vi "QuickTester.vi"() -> ()   [LabVIEW 2018]
uses:
  Real-Time/Control Algorithm/Control Algorithm Selection.ctl
  <vilib>/userdefined/High Color/nirio_resource_hc.ctl
  <vilib>/Simulation/Scripting/Companion Diagram/SimConfigNode/SimParams.ctl
  <vilib>/Simulation/Scripting/Companion Diagram/SimConfigNode/_simSolvers.ctl
  <vilib>/Simulation/Implementation/Shared/SIMSCR Execution Mode.ctl
  <vilib>/Platform/TimedLoop/XDataNode/timing_clust.ctl
  <vilib>/Platform/TimedLoop/XDataNode/nitl_modes.ctl
  <vilib>/Platform/TimedLoop/XDataNode/wakeup.ctl
  <vilib>/Simulation/Param Hierarchy/Typedefs/SIMPH Param Control Actions.ctl
  <vilib>/Simulation/Implementation/Shared/NILVSim_ParamChanged.vi
  <vilib>/Simulation/Implementation/Shared/NILVSim_FinishedLate.vi
  <vilib>/Simulation/Implementation/Shared/NILVSIM_BeginStep.vi
  <vilib>/Simulation/DiscreteLinear/Implementation/NILVSim Discrete State Space Direct.llb/SIM Discrete State Space Direct (MIMO).vi
  <vilib>/Simulation/Utility/Implementation/SIM Halt.vi
  <vilib>/Simulation/DiscreteLinear/Implementation/NILVSim Discrete Delay.llb/NILVSim Discrete Delay Buffered Distributor (scalar).vi
  <vilib>/Simulation/DiscreteLinear/Implementation/NILVSim Discrete Delay.llb/NILVSim Discrete Delay Buffered Collector (scalar).vi
  <vilib>/Simulation/Implementation/Shared/NILVSim_Manager.vi
  <vilib>/Utility/error.llb/Clear Errors.vi
  <vilib>/Simulation/Implementation/Shared/NILVSim_FinalizeModel.vi
  <vilib>/Simulation/Implementation/Shared/SIM Unbundle Sim Info.vi
  <vilib>/Simulation/Implementation/Shared/SIMSH Read Queue.vi
  <vilib>/Simulation/Implementation/Shared/NILVSim_Initialize.vi
  Real-Time/RT-FPGA Interface API/Read Tank Levels.vi
  <vilib>/Simulation/Utility/Implementation/NILVSim Get Time and IsAcceptedStep.vi
  <vilib>/Simulation/Implementation/Shared/NILVSim_GetModelError.vi
  <vilib>/Simulation/Implementation/Shared/SIM Bundle Sim Info.vi
  <vilib>/Simulation/Scripting/Companion Diagram/SimConfigNode/SimDog.xnode
  <vilib>/Platform/TimedLoop/XDataNode/XDataNode.xnode
  <vilib>/Simulation/Implementation/XNodeFramework/SimXNode/SimX.xnode
  Real-Time/RT-FPGA Interface API/RT-FPGA Interface API.lvlib
  <vilib>/Simulation/DiscreteLinear/Implementation/NILVSim Discrete Delay.llb/SIM Discrete Delay Buffered (scalar).vi
  <vilib>/Platform/TimedLoop/XDataNode/XDNodeRunTimeDep.lvlib
  <vilib>/Simulation/Implementation/Shared/NI_SIM_Implementation.lvlib
panel:
  out "coerced(x)":dbl[](array[numeric])
  in  "Halt?":bool
  out "Tanks levels":dbl[](array[numeric])
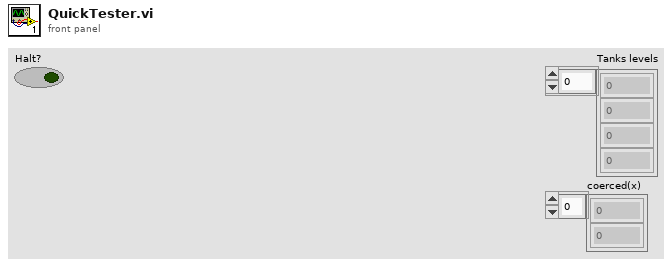
[diagram p1: front panel]
types:
  T1 = typedef "nirio_resource_hc.ctl" = tag
  T2 = typedef "Control Algorithm Selection.ctl" = enum16{"LQG-LTR", "Hinf"}
  T3 = cluster{"Plant model":cluster{"A":dbl[][], "B":dbl[][], "C":dbl[][], "D":dbl[][]}, "K robust control":cluster{"A":dbl[][], "B":dbl[][], "C":dbl[][], "D":dbl[][]}, "K w1":cluster{"A":dbl[][], "B":dbl[][], "C":dbl[][], "D":dbl[][]}, "K w2":cluster{"A":dbl[][], "B":dbl[][], "C":dbl[][], "D":dbl[][]}, "Sample period":dbl, "Control Algorithm selector":T2}
  T4 = cluster{"A":dbl[][], "B":dbl[][], "C":dbl[][], "D":dbl[][]}
  T5 = typedef "RT-FPGA Interface API.lvlib/FPGA ref.ctl" = refnum<k20>
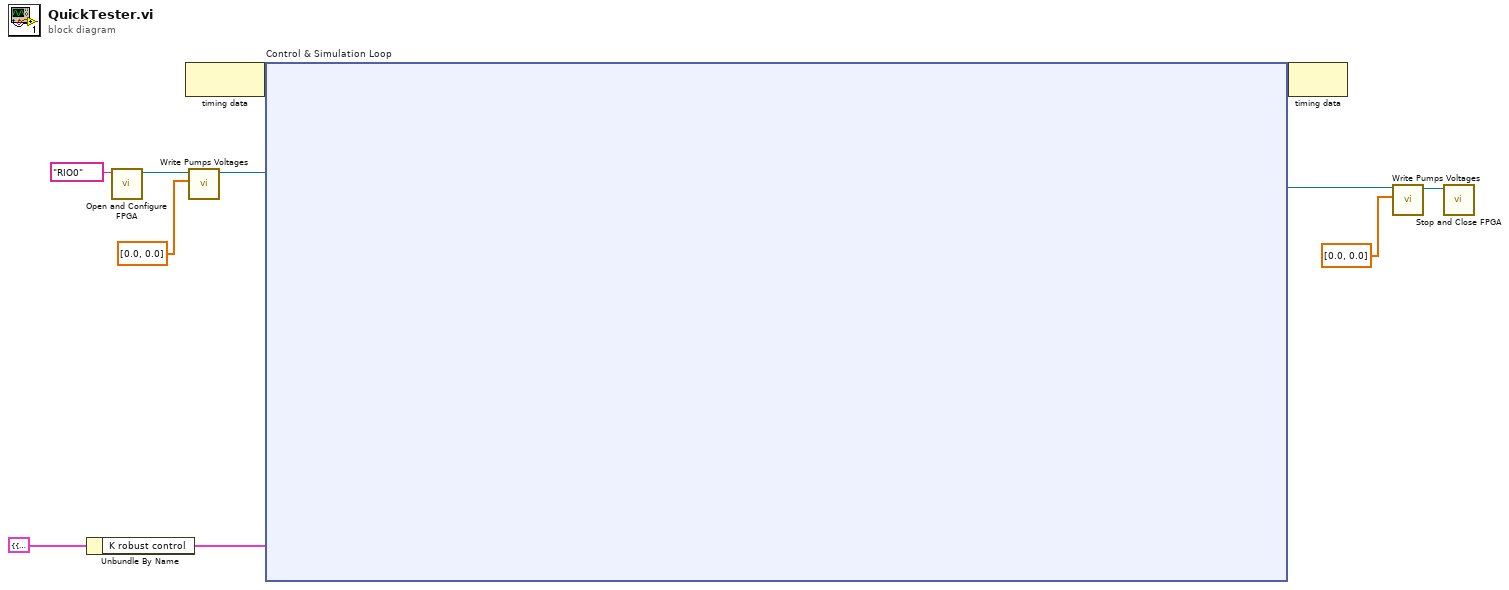
[diagram p0: block diagram]
diagram:
  n1 = Unbundle By Name(T3 {"Plant model"={"A"=[[-0.0334957, -0.745077, 0.0, 0.0], [0.745077, -0.0334957, 0.0, 0.0], [0.0, 0.0, 0.998593, 0.0], [0.0, 0.0, 0.0, 0.999334]], "B"=[[0.0638893, 0.0367221], [-0.01090059999999999, 0.0556748], [-0.00041721299999999, -1.547179999999e-05], [-0.00018019699999999, -0.00029937799999999]], "C"=[[-0.328419, -0.444393, 1.53754, -17.7295], [-1.28311, 1.32663, -12.9599, -8.5944]], "D"=[[0.0, 0.0], [0.0, 0.0]]}, "K robust control"={"A"=[[1.01599225076081, -1.5464195638756957, 0.15008465042516594, 0.5233292387133978], [0.04714525747524132, 0.14202756491251597, 0.16227009350481245, 0.3876921910923838], [0.04049870396502312, 0.7803474794750767, 0.6176248348433869, 1.4521263698431817], [8.5413449654e-07, -1.223762977532e-05, -1.157035082417e-05, -1.872201696223e-05]], "B"=[[-0.7479587101827235, -0.1793072086301349], [0.4769541880187386, -0.16571719620940878], [0.12803125046514824, -0.627049937730735], [-2.3692579782e-06, -0.456788973005955]], "C"=[[-0.03434480192684553, -0.6614285827425661, 0.2484472601052279, -1.6157674242426954], [-0.03745615785409984, 0.9266247553304973, -0.13853798436075038, 0.8450028566893902]], "D"=[[-0.36715050969228213, 0.10880464377707916], [-0.16776083785670542, 0.7443632894048002]]}, "K w1"={"A"=[[1.0, 0.0], [0.0, 1.0]], "B"=[[0.25, 0.0], [0.0, 0.25]], "C"=[[0.3999999999999999, 0.0], [0.0, 0.3999999999999999]], "D"=[[1.0, 0.0], [0.0, 1.0]]}, "K w2"={"A"=[], "B"=[], "C"=[], "D"=[]}, "Sample period"=0.1, "Control Algorithm selector"=enum."LQG-LTR"} ("Controllers out 2")) -> ("K robust control"=w8:T4)
  n2 = call "Open and Configure FPGA.vi"("resource name"=T1 "RIO0") -> ("FPGA VI Reference Out"=w6:T5)  [unwired: 9 in, 1 out]
  n3 = node-c288() -> (w11:variant)  [unwired: 1 in]
  n4 = call "Write Pumps Voltages.vi"("Pumps Voltages"=dbl[] [0.0, 0.0], "FPGA VI Reference In"=w6) -> ("FPGA VI Reference Out"=w5:T5)  [unwired: 8 in, 1 out]
  n5 = node-c254 "Control & Simulation Loop"(w11, w8, w5) -> (w10:variant, w2:T5)
  n6 = node-c288(w10) -> ()  [unwired: 1 out]
  n7 = call "Write Pumps Voltages.vi"("Pumps Voltages"=dbl[] [0.0, 0.0], "FPGA VI Reference In"=w2) -> ("FPGA VI Reference Out"=w1:T5)  [unwired: 8 in, 1 out]
  n8 = call "Stop and Close FPGA.vi"("FPGA VI Reference In"=w1) -> ()  [unwired: 10 in, 1 out]
